vi "S2DS_GW (SubVI).vi"(7 "Value to write":dbl, 8 "error in (no error)":errorcluster, 10 "GW1 Command format":string, 11 "VISA Refnum in":refnum<visa-resource-name>) -> (0 "error out":errorcluster)   [LabVIEW 2025]
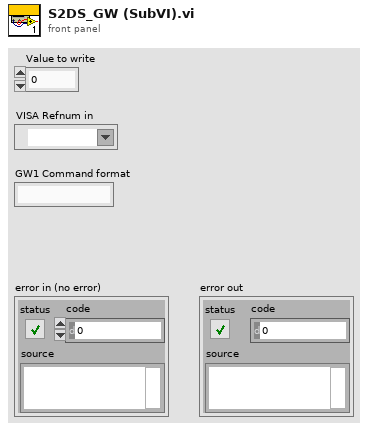
[diagram p1: front panel]
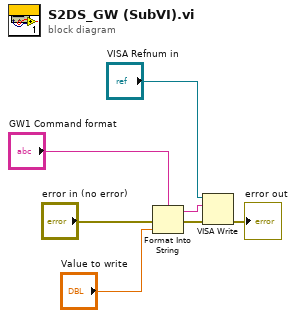
[diagram p0: block diagram]
diagram:
  n1 = Format Into String(format string="GW1 Command format", error in="error in (no error)", "Value to write") -> (resulting string=w3:string, error out=w1:errorcluster)  [unwired: 1 in]
  n2 = VISA Write(VISA resource name="VISA Refnum in", write buffer=w3, error in (no error)=w1) -> (error out=→"error out":errorcluster)  [unwired: 2 out]
